vi "AcquisitionStatus.vi"(8 "error in (no error)":errorcluster, 10 "MaxTime(5000mS)":u32=5000, 11 "Keysight44xx in":refnum<class "Keysight44xx.lvclass">) -> (0 "error out":errorcluster, 2 "Acquisition Status":i32, 3 "Keysight44xx out":refnum<class "Keysight44xx.lvclass">)   [LabVIEW 2018, in "SpecAnPlugins.lvlib" / "Keysight44xx.lvclass"]
doc: "This function determines and returns the status of an acquisition."
uses:
  Keysight44xx.lvclass
  C:/Users/ico/Documents/Projects/NistPluggableModules/SpecAn/SpecAnPlugins/SpecAnBaseClass/SpecAnBase.lvclass
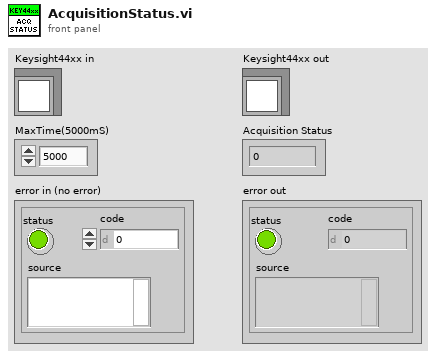
[diagram p1: front panel]
types:
  T1 = typedef "SpecAnPlugins.lvlib/SpecAnBase.lvclass/Acquisition.ctl" = cluster{"Handle":string, "Connected":bool, "Enabled":bool, "SweepModeContinuous":bool, "NumberOfSweeps":i32, "DetectorTypeAuto":bool, "DetectorType":i32, "VerticalScale":i32, "MaximumTime(seconds)":dbl}
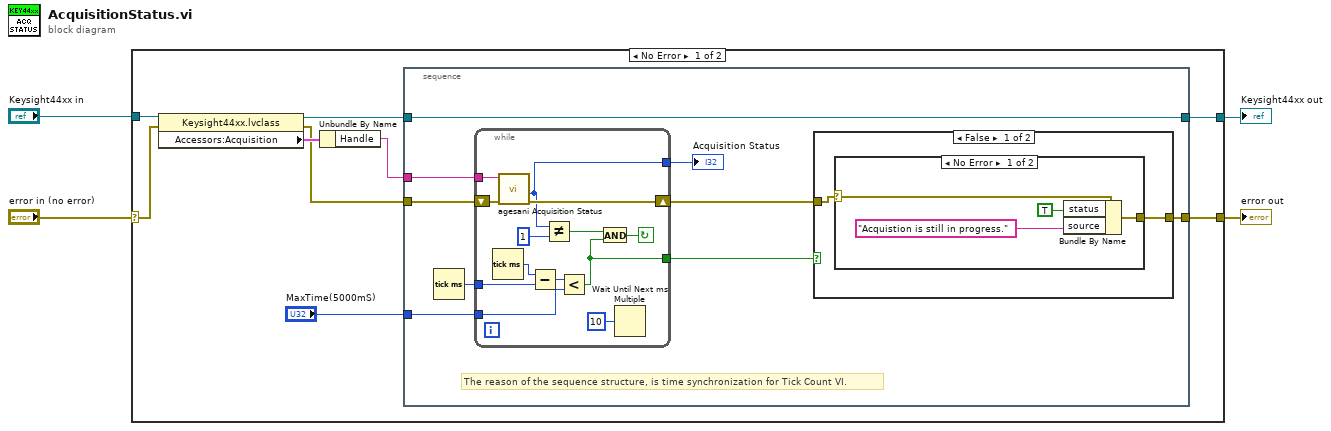
[diagram p0: block diagram]
diagram:
  n1 = case shown="No Error" "error in (no error)" {
    selector: "error in (no error)" -> [w12 w44]
    tunnel: "Keysight44xx in" -> [w13 w45]
    tunnel: [w8 w45] -> w2
    tunnel: [w6 w44] -> w1
    frame No Error {
      n2 = property class="Keysight44xx.lvclass"(reference=w13, error in=w12) -> (reference out=w9:refnum<class "Keysight44xx.lvclass">, error out=w10:errorcluster, "Accessors:Acquisition"=w11:T1)
      n3 = Unbundle By Name(w11) -> ("Handle"=w7:string)
      n4 = stacked-sequence {
        tunnel: w10 -> [w22]
        tunnel: w7 -> [w21]
        tunnel: [w17] -> w6
        tunnel: w9 -> [w16]
        tunnel: [w16] -> w8
        tunnel: "MaxTime(5000mS)" -> [w15]
        frame #0 {
          # "The reason of the sequence structure, is time synchronization for Tick Count VI."
          n5 = Tick Count (ms)() -> (millisecond timer value=w20:u32)
          n6 = while {
            shift-right: [w32] -> w18
            shift-left: w22 -> [w33]
            tunnel: w21 -> [w34]
            tunnel: w20 -> [w40]
            tunnel: w15 -> [w38]
            tunnel: [w35] -> w19
            tunnel: [w31] -> w14
            stop <- w37 continue-if-true
            n7 = Tick Count (ms)() -> (millisecond timer value=w41:u32)
            n8 = call <instrlib>:"agesani Acquisition Status.vi"("error in (no error)"=w33, "instrument handle"=w34) -> ("error out"=w32:errorcluster, "acquisition status"=w31:i32)  [unwired: 7 in, 1 out]
            n9 = Subtract(x=w41, y=w40) -> (x-y=w39:u32)
            n10 = Not Equal?(x=w31, y=1) -> (x != y?=w36:bool)
            n11 = Less?(x=w39, y=w38) -> (x < y?=w35:bool)
            n12 = And(x=w36, y=w35) -> (x .and. y?=w37:bool)
            n13 = Wait Until Next ms Multiple(millisecond multiple=u32 10) -> ()  [unwired: 1 out]
          }
          "Acquisition Status" <- w14
          n14 = case shown="False" w19 {
            tunnel: w18 -> [w24 w30]
            tunnel: [w23 w30] -> w17
            frame False {
              n15 = case shown="No Error" w24 {
                selector: w24 -> [w28 w29]
                tunnel: [w27 w29] -> w23
                frame No Error {
                  n16 = Bundle By Name(cluster=w28, "status"=TRUE, "source"="Acquistion is still in progress.") -> (w27:errorcluster)
                }
                frame Error {
                }
              }
            }
            frame True {
            }
          }
        }
      }
    }
    frame Error {
    }
  }
  "error out" <- w1
  "Keysight44xx out" <- w2
